vi "P_D_SQR+COL.vi"() -> ()   [LabVIEW 2017]
uses:
  <vilib>/vision/Image Controls.llb/IMAQ Image.ctl
  <vilib>/vision/Pattern Matching.llb/IMAQ GM Match Report.ctl
panel:
  in  "Stop Button":bool
  out "Class (Particle Classification 1)":string
  in  "ROI":T1={"Global Rectangle"=[0, 0, 638, 479], "Contours"=[{"ID"=enum."External", "Type"=3, "Coordinates"=[0, 0, 638, 479]}]} {"Contours"."Type" items=["No Selection", "Point", "Line", "Rectangle", "Oval", "Polygon", "Freehand Region", "Annulus", "Unused2", "Unused3", "Broken Line", "Freehand Line", "Rotated Rectangle"]}
  out "y0":i32
  out "x0":i32
  out "x1":i32
  out "y1":i32
  out "Scale":sgl
  in  "y":sgl=1.0
  out "Number of Matches (Geometric Matching 1)":i32
  out "Calibrated Matches (Geometric Matching 1)":T2[](array[typedef]) {"Correlation Score" format="%.2f"; "Target Template Curve Score" format="%.2f"; "Template Target Curve Score" format="%.2f"; "Bounding Box"."y" format="%.2f"; "Bounding Box"."x" format="%.2f"; "Position"."y" format="%.2f"; "Position"."x" format="%.2f"; "Score" format="%.2f"; "Scale" format="%.2f"; "Angle" format="%.2f"; "Occlusion %" format="%.2f"}
  out "analyzed Image":T3
  out "error out":errorcluster
  out "web cam Image":T3(plugin-control)
  in  "error in":errorcluster
  in  "Stop (F)":bool
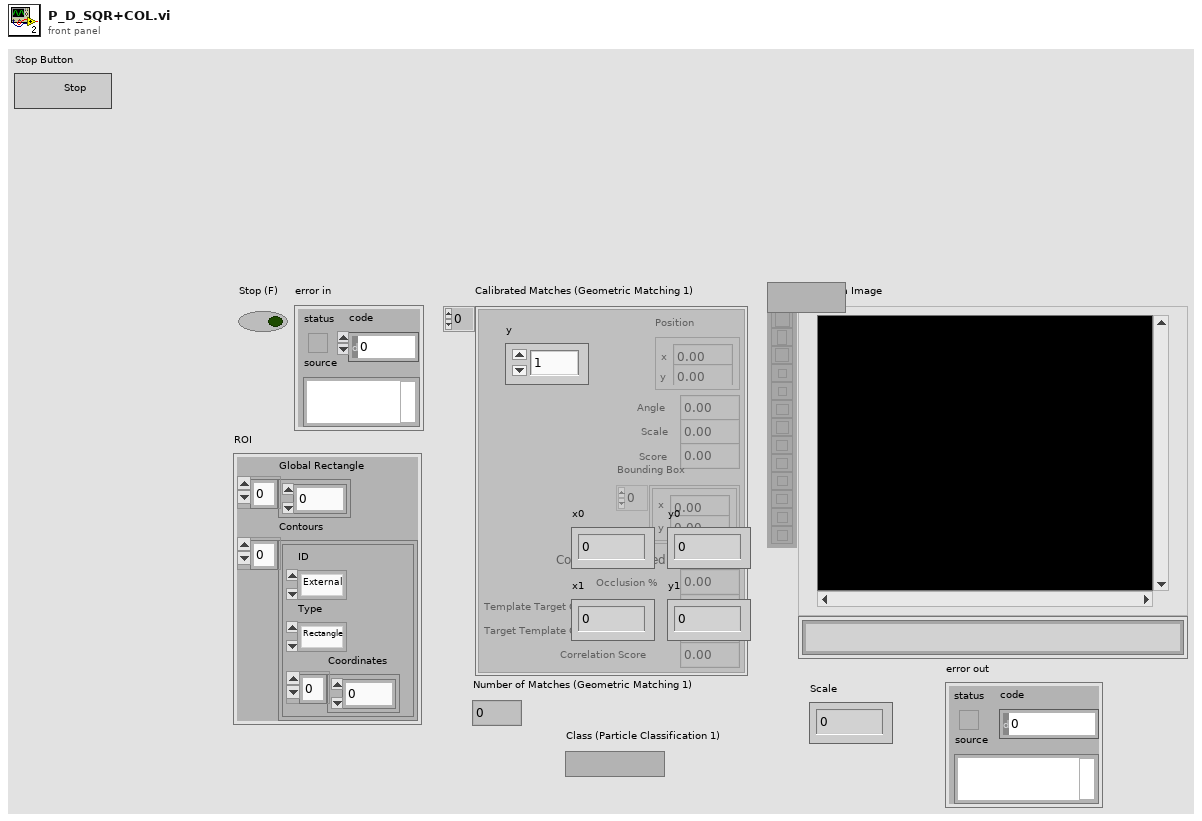
[diagram p1: front panel]
types:
  T1 = cluster{"Global Rectangle":i32[], "Contours":cluster{"ID":enum32{"External", "Internal"}, "Type":u32, "Coordinates":i32[]}[]}
  T2 = typedef "IMAQ GM Match Report.ctl" = cluster{"Position":cluster{"x":sgl, "y":sgl}, "Angle":sgl, "Scale":sgl, "Score":sgl, "Bounding Box":cluster{"x":sgl, "y":sgl}[], "Contrast Reversed":bool, "Occlusion %":sgl, "Template Target Curve Score":sgl, "Target Template Curve Score":sgl, "Correlation Score":sgl}
  T3 = typedef "IMAQ Image.ctl" = refnum<image>
  T4 = cluster{"ID":enum32{"External", "Internal"}, "Type":u32, "Coordinates":i32[]}[]
  T5 = cluster{"ID":enum32{"External", "Internal"}, "Type":u32, "Coordinates":i32[]}
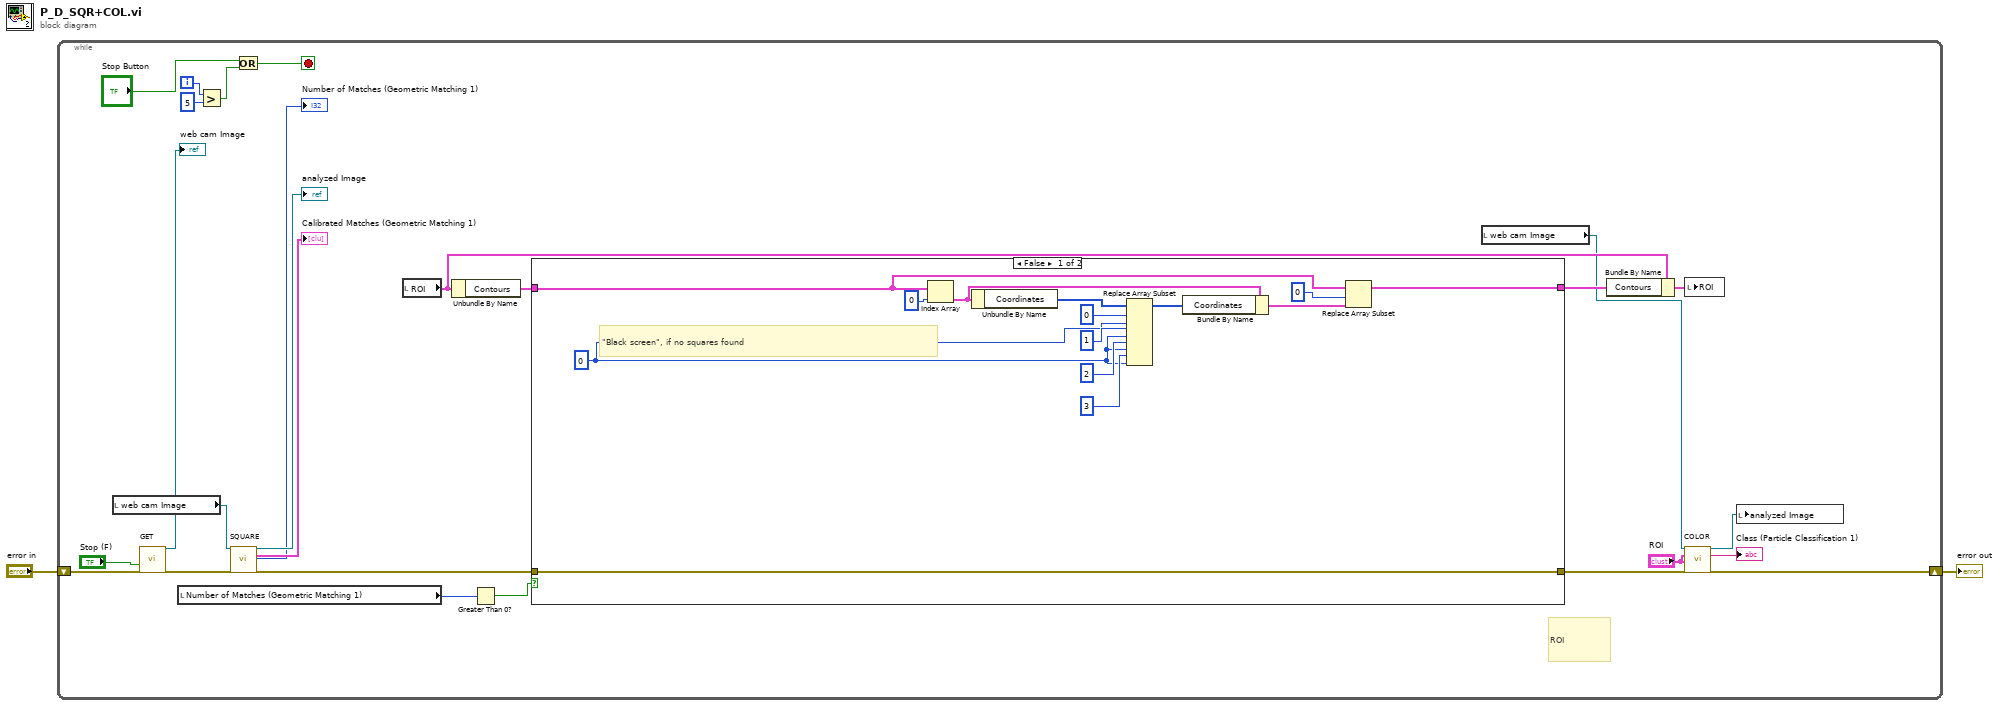
[diagram p0: block diagram]
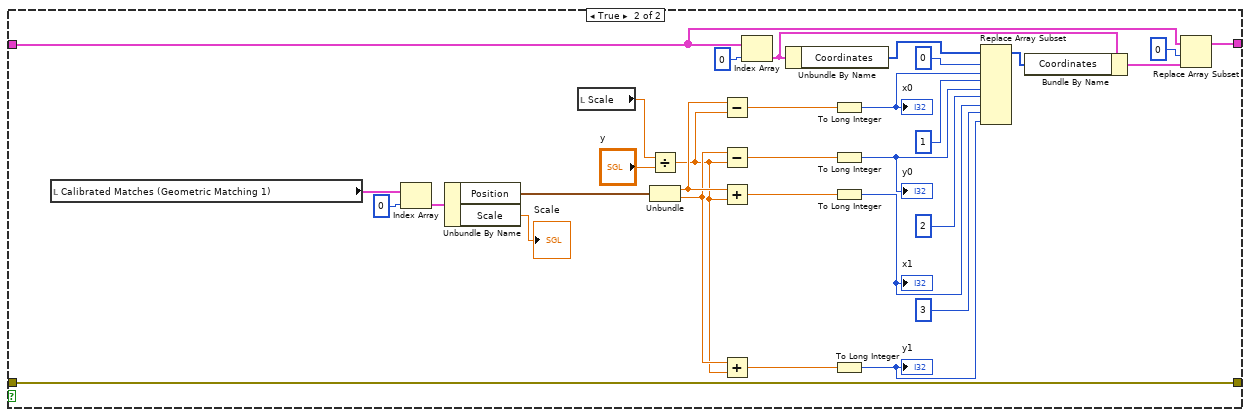
[diagram p2: hidden frame]
diagram:
  n1 = while {
    shift-right: [w12] -> w1
    shift-left: "error in" -> [w27]
    i -> [w4]
    stop <- w6 stop-if-true
    # "ROI"
    n2 = local read "web cam Image"() -> (w25:T3)
    n3 = call "GET"("Stop (F)"="Stop (F)", "error in"=w27) -> ("Image Out"=→"web cam Image":T3, "error out"=w24:errorcluster)  [unwired: 22 in, 2 out]
    n4 = local read "Number of Matches (Geometric Matching 1)"() -> (w19:i32)
    n5 = Greater?(x=w4, y=5) -> (0:w3:bool)
    n6 = call "SQUARE"("Image In"=w25, "error in"=w24) -> ("Image Out"=→"analyzed Image":T3, "Calibrated Matches (Geometric Matching 1)"=→"Calibrated Matches (Geometric Matching 1)":T2[], "Number of Matches (Geometric Matching 1)"=→"Number of Matches (Geometric Matching 1)":i32, "error out"=w8:errorcluster)  [unwired: 22 in]
    n7 = Or(x="Stop Button", y=w3) -> (x .or. y?=w6:bool)
    n8 = local read "ROI"() -> (w15:T1)
    n9 = Unbundle By Name(w15) -> ("Contours"=w17:T4)
    n10 = Greater Than 0?(x=w19) -> (x > 0?=w20:bool)
    n11 = case shown="False" w20 {
      tunnel: [w30 w44] -> w14
      tunnel: w17 -> [w31 w45]
      tunnel: [w29 w43] -> w9
      tunnel: w8 -> [w29 w43]
      frame False {
        w32 = 0 ("index")
        # "\"Black screen\", if no squares found"
        n12 = Index Array(array=w31, index=0) -> (element=w40:T5)
        n13 = Unbundle By Name(w40) -> ("Coordinates"=w39:i32[])
        n14 = Replace Array Subset(array=w39, new element #1=w32, index #1=0 ("index"), new element #2=w32, index #2=1 ("index"), new element #3=w32, index #3=2 ("index"), new element #4=w32, index #4=3 ("index")) -> (w41:i32[])
        n15 = Bundle By Name(cluster=w40, "Coordinates"=w41) -> (w42:T5)
        n16 = Replace Array Subset(array=w31, new element=w42, index=0) -> (w30:T4)
      }
      frame True {
        n17 = local read "Calibrated Matches (Geometric Matching 1)"() -> (w73:T2[])
        n18 = Index Array(array=w73, index=0) -> (element=w71:T2)
        n19 = Unbundle By Name(w71) -> ("Position"=w70:cluster{"x":sgl, "y":sgl}, "Scale"=→"Scale":sgl)
        n20 = local read "Scale"() -> (w48:sgl)
        n21 = Divide(x=w48, y="y") -> (x/y=w47:sgl)
        n22 = Unbundle(w70) -> ("x"=w67:sgl, "y"=w66:sgl)
        n23 = Subtract(x=w67, y=w47) -> (x-y=w65:sgl)
        n24 = Subtract(x=w66, y=w47) -> (x-y=w64:sgl)
        n25 = Add(x=w67, y=w47) -> (x+y=w62:sgl)
        n26 = Add(x=w66, y=w47) -> (x+y=w63:sgl)
        n27 = Index Array(array=w45, index=0) -> (element=w59:T5)
        n28 = Unbundle By Name(w59) -> ("Coordinates"=w61:i32[])
        n29 = To Long Integer(number=w65) -> (32bit integer=w56:i32)
        "x0" <- w56
        n30 = To Long Integer(number=w64) -> (32bit integer=w55:i32)
        "y0" <- w55
        n31 = To Long Integer(number=w62) -> (32bit integer=w54:i32)
        "x1" <- w54
        n32 = To Long Integer(number=w63) -> (32bit integer=w53:i32)
        "y1" <- w53
        n33 = Replace Array Subset(array=w61, new element #1=w56, index #1=0 ("index"), new element #2=w55, index #2=1 ("index"), new element #3=w54, index #3=2 ("index"), new element #4=w53, index #4=3 ("index")) -> (w58:i32[])
        n34 = Bundle By Name(cluster=w59, "Coordinates"=w58) -> (w57:T5)
        n35 = Replace Array Subset(array=w45, new element=w57, index=0) -> (w44:T4)
      }
    }
    n36 = local read "web cam Image"() -> (w10:T3)
    n37 = Bundle By Name(cluster=w15, "Contours"=w14) -> (w16:T1)
    n38 = local write "ROI"(w16) -> ()
    n39 = call "COLOR"("Image In"=w10, "ROI Descriptor (Image Mask 1)"="ROI", "ROI Descriptor (Particle Classification 1)"="ROI", "error in"=w9) -> ("Image Out"=w11:T3, "Class (Particle Classification 1)"=→"Class (Particle Classification 1)":string, "error out"=w12:errorcluster)  [unwired: 21 in]
    n40 = local write "analyzed Image"(w11) -> ()
  }
  "error out" <- w1
